vi "Practica 4.vi"() -> ()   [LabVIEW 2018]
uses:
  <vilib>/LabVIEW Interface for Arduino/Type Defs/Pin Mode.ctl
  <vilib>/LabVIEW Interface for Arduino/LabVIEW Interface for Arduino.lvlib
panel:
  out "Medida A0":dbl(knob) scale=0.0..10.0
  in  "stop":bool
  out "LED 8":bool
  in  "Pin 8":bool
  out "Salida":dbl(slide) scale=0.0..255.0
  in  "Valor analogico":dbl(knob) scale=0.0..255.0
  # "Practica 4: Lectura Escritura de valores"
  # "Gobierno Salida Digital Pin 8"
  # "Valor enviado a la salida PWM PIN 3"
  # "Valor leido Entrada Analogica A0"
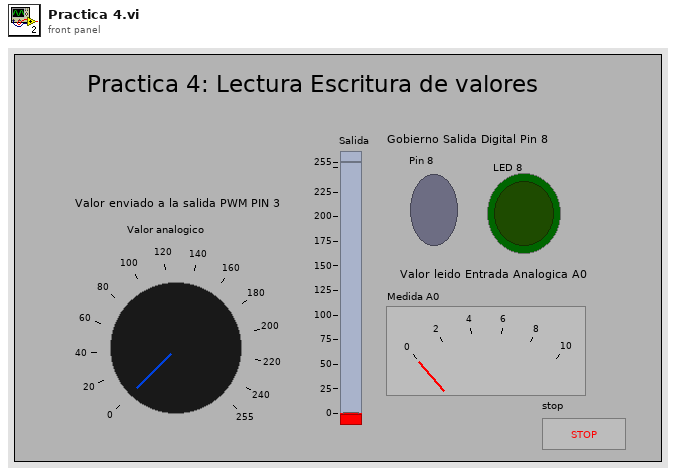
[diagram p1: front panel]
types:
  T1 = typedef "LabVIEW Interface for Arduino.lvlib/Pin Mode.ctl" = enum8{"Input", "Output"}
  T2 = typedef "LabVIEW Interface for Arduino.lvlib/Arduino Resource.ctl" = cluster{"VISA resource":refnum<visa-resource-name>, "Board Type":T3, "Connection Type":enum8{"USB / Serial"}, "Bytes Per Packet (15)":u8}
  T3 = typedef "LabVIEW Interface for Arduino.lvlib/Board Type.ctl" = enum16{"Uno", "Dimuelanove w/Atmega 328", "Mega 2560"}
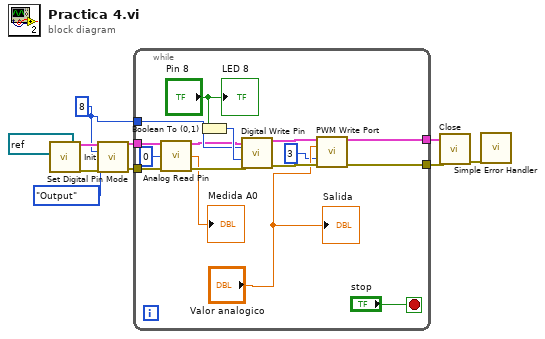
[diagram p0: block diagram]
diagram:
  w3 = u8 8 ("Digital I/O Pin")
  n1 = call <vilib>:"Init.vi"("VISA resource"=refnum<visa-resource-name> "COM9") -> ("Arduino Resource"=w10:T2, "error out"=w9:errorcluster)  [unwired: 17 in]
  n2 = call <vilib>:"Set Digital Pin Mode.vi"("Arduino Resource"=w10, "Digital I/O Pin"=w3, "Pin Mode (Input)"=Pin_Mode."Output", "error in"=w9) -> ("Arduino Resource"=w8:T2, "error out"=w7:errorcluster)  [unwired: 10 in]
  n3 = while {
    tunnel: w8 -> [w12]
    tunnel: w7 -> [w11]
    tunnel: [w23] -> w5
    tunnel: [w22] -> w4
    tunnel: w3 -> [w19]
    stop <- "stop" stop-if-true
    n4 = call <vilib>:"Analog Read Pin.vi"("Arduino Resource"=w12, "Analog Input Pin (0)"=u8 0 ("Digital I/O Pin (0)"), "error in"=w11) -> ("Arduino Resource"=w13:T2, "Voltage"=→"Medida A0":dbl, "error out"=w15:errorcluster)  [unwired: 10 in]
    n5 = Boolean To (0,1)(Boolean="Pin 8") -> (0, 1=w20:i16)
    n6 = call <vilib>:"Digital Write Pin.vi"("Arduino Resource"=w13, "Digital I/O Pin (0)"=w19, "Value (0)"=w20, "error in"=w15) -> ("Arduino Resource"=w25:T2, "error out"=w24:errorcluster)  [unwired: 10 in]
    n7 = call <vilib>:"PWM Write Port.vi"("Arduino Resource"=w25, "PWM 0 (0-255)"="Valor analogico", "PWM 2 (0-255)"=u8 3, "error in"=w24) -> ("Arduino Resource"=w23:T2, "error out"=w22:errorcluster)  [unwired: 9 in, 1 out]
    "Salida" <- "Valor analogico"
    "LED 8" <- "Pin 8"
  }
  n8 = call <vilib>:"Close.vi"("Arduino Resource"=w5, "error in"=w4) -> ("error out"=w6:errorcluster)  [unwired: 13 in]
  n9 = call <vilib>:"Simple Error Handler.vi"("error in (no error)"=w6) -> ()  [unwired: 4 in, 5 out]
